vi "Is Window Visible.vi"(8 "error in (no error)":errorcluster, 11 "WindowHandleIn":T1) -> (0 "error out":errorcluster, 2 "WindowVisible":bool, 3 "WindowHandle":T1)   [LabVIEW 2015]
uses:
  user32.dll
panel:
  in  "WindowHandle 2":T1
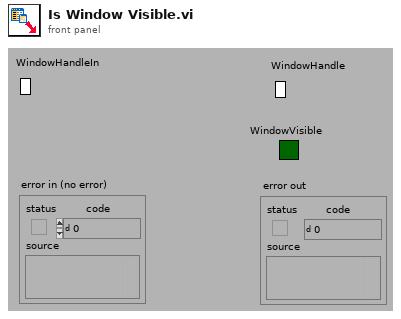
[diagram p1: front panel]
types:
  T1 = typedef "WindowHandle" = refnum<k1>
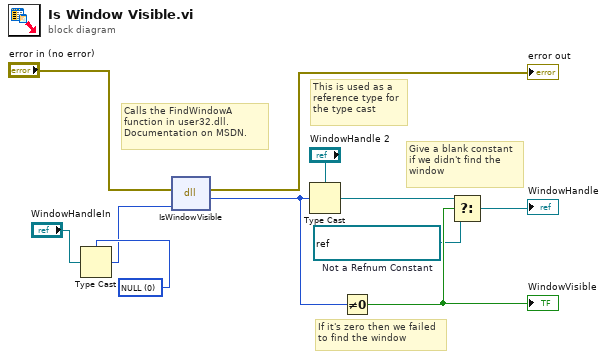
[diagram p0: block diagram]
diagram:
  w3 = u32 0 items=["NULL"]
  w6 = refnum<k0> refnum  # Not a Refnum Constant
  # "If it's zero then we failed\nto find the window"
  # "Give a blank constant\nif we didn't find the\nwindow"
  # "This is used as a \nreference type for\nthe type cast"
  # "Calls the FindWindowA\nfunction in user32.dll.\nDocumentation on MSDN."
  n1 = Type Cast(type=w3, x="WindowHandleIn") -> (*(type *) &x=w1:u32)
  n2 = dll-call lib="user32.dll" fn="IsWindowVisible"(error in="error in (no error)", "hWnd"=w1) -> (error out=→"error out":errorcluster, "return type"=w10:u32)  [unwired: 3 in, 1 out]
  n3 = Type Cast(type="WindowHandle 2", x=w10) -> (*(type *) &x=w9:T1)
  n4 = Not Equal To 0?(x=w10) -> (x != 0?=w8:bool)
  "WindowVisible" <- w8
  n5 = Select(t=w9, s=w8, f=w6) -> (s? t:f=→"WindowHandle":T1)
